vi "Write StrEdit.vi"(8 "error in (no error)":errorcluster, 10 "StrEdit":refnum<vi>, 11 "MCListbox View in":refnum<class "MCListbox View.lvclass">) -> (0 "error out":errorcluster, 3 "MCListbox View out":refnum<class "MCListbox View.lvclass">)   [LabVIEW 2013, in "SET Project Editor.lvlib" / "MCListbox View.lvclass"]
uses:
  MCListbox View.lvclass
  MCListbox View.lvclass/MCListbox View.ctl
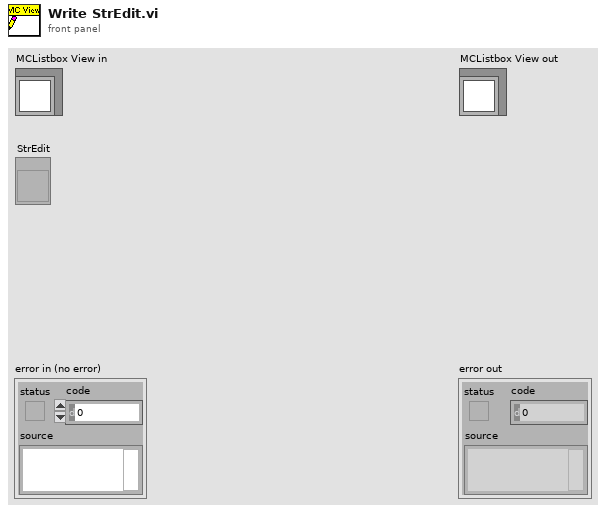
[diagram p1: front panel]
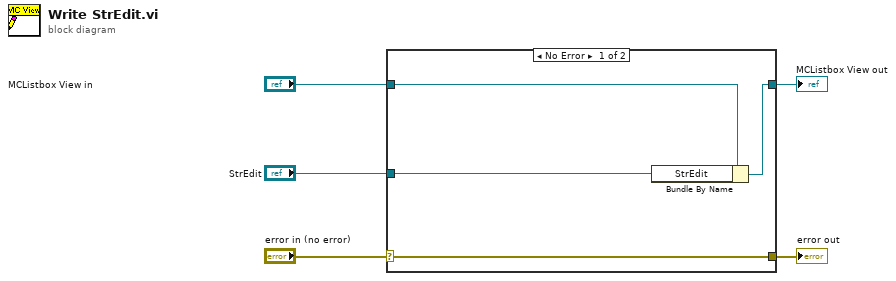
[diagram p0: block diagram]
diagram:
  n1 = case shown="No Error" "error in (no error)" {
    selector: "error in (no error)" -> [w9 w10]
    tunnel: [w9 w10] -> w4
    tunnel: [w7 w11] -> w2
    tunnel: "MCListbox View in" -> [w8 w11]
    tunnel: "StrEdit" -> [w6 _]
    frame No Error {
      n2 = Bundle By Name(cluster=w8, "StrEdit"=w6) -> (w7:refnum<class "MCListbox View.lvclass">)
    }
    frame Error {
    }
  }
  "error out" <- w4
  "MCListbox View out" <- w2
